vi "UI_Prepare_Report.vi"(8 "error in (no error)":errorcluster caption="entrée d'erreur (pas d'erreur)", 10 "UI Status":T4, 11 "QMH UI Cluster":T1) -> (0 "error out":errorcluster caption="sortie d'erreur", 2 "Variant":variant, 3 "QMH UI Cluster":T1)   [LabVIEW 2015]
uses:
  controls/QMH_UI_Cluster.ctl
  controls/QMH_UI_References.ctl
  controls/QMH_UI_Report.ctl
  controls/QMH_UI_Command.ctl
  controls/QMH_ICR_Command.ctl
  controls/QMH_Status.ctl
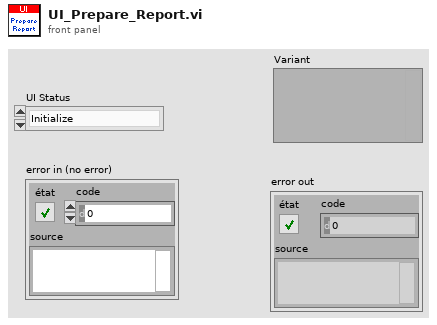
[diagram p1: front panel]
types:
  T1 = typedef "QMH_UI_Cluster.ctl" = cluster{"QMH UI References":T2, "QMH UI Report":T3}
  T2 = typedef "QMH_UI_References.ctl" = cluster{"Refnum Load":refnum<vi>, "Refnum Save":refnum<vi>, "Refnum Start":refnum<vi>, "Refnum Stop":refnum<vi>, "Refnum Exit":refnum<vi>, "Refnum Tabs":refnum<vi>, "Refnum SPECTRUM":refnum<vi>, "Refnum EXPERIMENT":refnum<vi>, "Refnum VOLTAGES":refnum<vi>, "Refnum SEQUENCE":refnum<vi>, "Refnum EXPERT":refnum<vi>, "Refnum CHANGE Experiment":refnum<vi>, "Refnum CHANGE Voltages":refnum<vi>, "Refnum CHANGE Sequence":refnum<vi>, "Refnum CHANGE Expert":refnum<vi>}
  T3 = typedef "QMH_UI_Report.ctl" = cluster{"UI Status":T4, "QLA Status":string, "ICR Status":T5, "QMH Status":T6}
  T4 = typedef "QMH_UI_Command.ctl" = enum16{"Initialize", "UI Load", "UI Save", "UI Change Experiment", "UI Change Voltages", "UI Change Sequence", "UI Change Expert", "Ready to Start", "UI Start", "UI Stop", "UI Exit", "Update Report", "Update ICR Report"}
  T5 = typedef "QMH_ICR_Command.ctl" = enum16{"Initialize", "Hardware Setup", "Waiting for Trigger", "Sequence Started", "Sequence Finished", "Writing Data", "Hardware Reset", "Exit"}
  T6 = typedef "QMH_Status.ctl" = enum16{"Init", "Loading", "Setup", "Ready to Start", "Started", "Idle"}
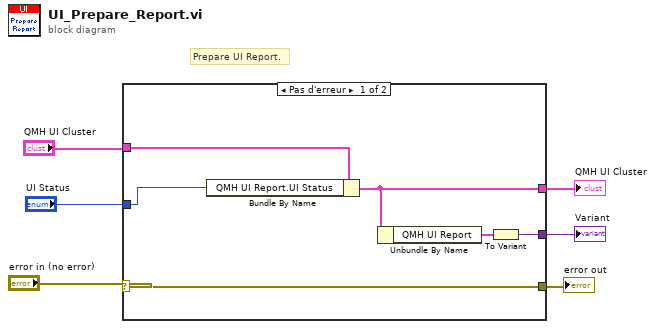
[diagram p0: block diagram]
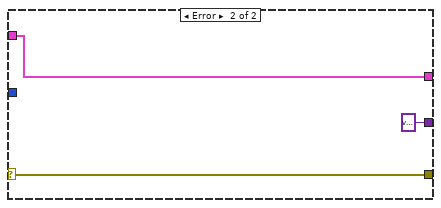
[diagram p2: hidden frame]
diagram:
  # "Prepare UI Report."
  n1 = case shown="Pas d'erreur" "error in (no error)" {
    selector: "error in (no error)" -> [w12 w15]
    tunnel: [w12 w15] -> w5
    tunnel: "QMH UI Cluster" -> [w11 w13]
    tunnel: "UI Status" -> [w7 _]
    tunnel: [w10 w13] -> w2
    tunnel: [w8 variant ("Variant")] -> w1
    frame No Error {
      n2 = Bundle By Name(cluster=w11, "QMH UI Report.UI Status"=w7) -> (w10:T1)
      n3 = Unbundle By Name(w10) -> ("QMH UI Report"=w9:T3)
      n4 = To Variant(anything=w9) -> (Variant=w8:variant)
    }
    frame Error {
    }
  }
  "error out" <- w5
  "QMH UI Cluster" <- w2
  "Variant" <- w1
